vi "DEN Unit Tests.vi"() -> ()   [LabVIEW 2018]
uses:
  <vilib>/rvi/DesktopExecutionNode/Execution/niFpgaDEN_Execute.vi
  <vilib>/rvi/DesktopExecutionNode/DesktopExecutionNode.xnode
panel:
  out "Readouts":u8[](array[numeric])
  in  "Commands":u8[](array[numeric])
  in  "Reads":u8[](array[numeric])
  out "Writes":u8[](array[numeric])
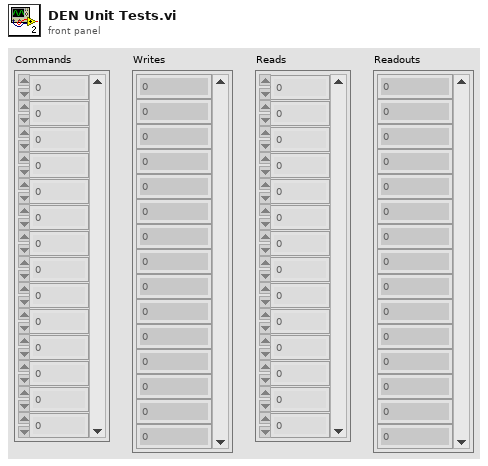
[diagram p1: front panel]
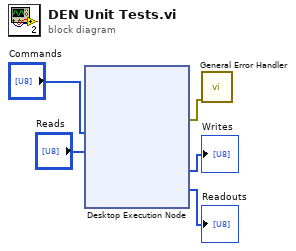
[diagram p0: block diagram]
diagram:
  n1 = xnode "Desktop Execution Node"("Commands"="Commands", "Reads"="Reads") -> ("Error Out"=w1:errorcluster, "Writes"=→"Writes":u8[], "Readouts"=→"Readouts":u8[])  [unwired: 1 in]
  n2 = call <vilib>:"General Error Handler.vi"("error in (no error)"=w1) -> ()  [unwired: 10 in, 5 out]
